vi "Z900_navX_Internal_StartLoop.vi"(8 "error in (no error)":errorcluster, 11 "navX Device":T1={"Interface"={"Protocol"=enum."SERIAL", "Update Rate (4Hz-60Hz)"=4, "navX Open TypeDef"=variant}, "Notify Packet"=refnum, "Loop VI Refnum"=refnum, "Ready to Close Occurrence Refnum"=refnum} {"Interface"."Update Rate (4Hz-60Hz)" min=4 max=60 step=1}) -> (0 "error out":errorcluster, 3 "navX Device":T1={"Interface"={"Protocol"=enum."SERIAL", "Update Rate (4Hz-60Hz)"=4, "navX Open TypeDef"=variant}, "Notify Packet"=refnum, "Loop VI Refnum"=refnum, "Ready to Close Occurrence Refnum"=refnum} {"Interface"."Update Rate (4Hz-60Hz)" min=4 max=60 step=1})   [LabVIEW 2016, in "navX Library v2.lvlib"]
doc: "This navX VI handles starting the background processing loop for the navX.\nTHIS VI SHOULD NOT BE CALLED BY THE USER!"
uses:
  navX Library v2.lvlib
  TypeDefs/Z900_navX_DeviceTypeDef.ctl
  TypeDefs/Z900_navX_ProtocolTypeDef.ctl
  TypeDefs/Z900_navX_NotifyPacketTypeDef.ctl
  TypeDefs/Z900_navX_ActionTypeDef.ctl
  Z900_navX_Internal_ProcessingLoop.vi
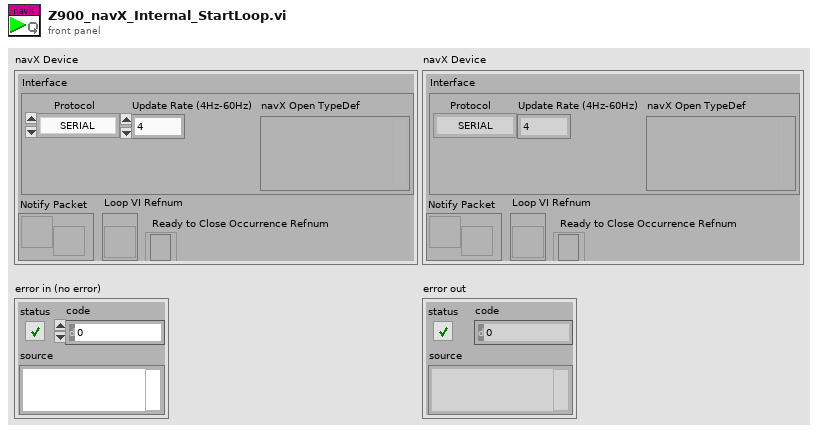
[diagram p1: front panel]
types:
  T1 = typedef "navX Library v2.lvlib/Z900_navX_DeviceTypeDef.ctl" = cluster{"Interface":cluster{"Protocol":T2, "Update Rate (4Hz-60Hz)":u8, "navX Open TypeDef":variant}, "Notify Packet":refnum<notifier>, "Loop VI Refnum":refnum<vi>, "Ready to Close Occurrence Refnum":refnum<k4>}
  T2 = typedef "navX Library v2.lvlib/Z900_navX_ProtocolTypeDef.ctl" = enum16{"SERIAL", "I2C", "SPI"}
  T3 = typedef "navX Library v2.lvlib/Z900_navX_NotifyPacketTypeDef.ctl" = cluster{"navX Action":T4, "Data":variant}
  T4 = typedef "navX Library v2.lvlib/Z900_navX_ActionTypeDef.ctl" = enum16{"None", "Halt", "Update Serial Protocol", "Zero-Yaw", "Zero-Displacement", "Zero-Velocity"}
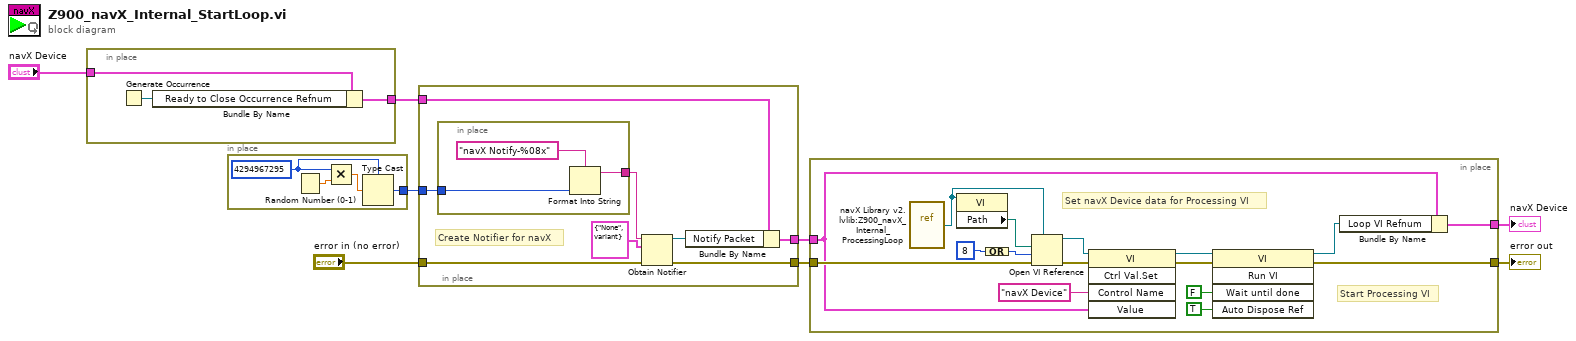
[diagram p0: block diagram]
diagram:
  n1 = in-place {
    in-place-border: "navX Device" -> [w11]
    in-place-border: [w9] -> w2
    n2 = Generate Occurrence() -> (w10:refnum<k4>)
    n3 = Bundle By Name(cluster=w11, "Ready to Close Occurrence Refnum"=w10) -> (w9:T1)
  }
  n4 = in-place {
    in-place-border: [w12] -> w8
    w14 = u32 4294967295
    n5 = Random Number (0-1)() -> (number: 0 to 1=w15:dbl)
    n6 = Multiply(x=w14, y=w15) -> (x*y=w13:dbl)
    n7 = Type Cast(type=w14, x=w13) -> (*(type *) &x=w12:u32)
  }
  n8 = in-place {
    in-place-border: w2 -> [w23]
    in-place-border: [w22] -> w5
    in-place-border: "error in (no error)" -> [w19]
    in-place-border: w8 -> [w17]
    in-place-border: [w16] -> w6
    # "Create Notifier for navX"
    n9 = in-place {
      in-place-border: [w25] -> w18
      in-place-border: w17 -> [w24]
      n10 = Format Into String(format string="navX Notify-%08x" ("name (unnamed)"), w24) -> (resulting string=w25:string)  [unwired: 2 in, 1 out]
    }
    n11 = Obtain Notifier(name (unnamed)=w18, notification data type=T3 {"navX Action"=enum."None", "Data"=variant} ("navX Notify Packet"), error in (no error)=w19) -> (notifier out=w21:refnum<notifier>, error out=w16:errorcluster)  [unwired: 1 in, 1 out]
    n12 = Bundle By Name(cluster=w23, "Notify Packet"=w21) -> (w22:T1)
  }
  n13 = in-place {
    in-place-border: w6 -> [w40]
    in-place-border: [w41] -> w4
    in-place-border: [w42] -> w3
    in-place-border: w5 -> [w39]
    # "Start Processing VI"
    # "Set navX Device data for Processing VI"
    n14 = vi-ref "navX Library v2.lvlib:Z900_navX_Internal_ProcessingLoop.vi"() -> (w28:refnum<vi>)
    n15 = property class="VI"(reference=w28) -> ("Path"=w37:path)  [unwired: 1 in, 2 out]
    n16 = Compound Arithmetic op=OR(8) -> (w38:i32)
    n17 = Open VI Reference(type specifier VI Refnum (for type only)=w28, vi path=w37, options=w38, error in (no error)=w40) -> (vi reference=w31:refnum<vi>, error out=w27:errorcluster)  [unwired: 2 in]
    n18 = invoke class="VI" method="Ctrl Val.Set"(reference=w31, error in=w27, "Control Name"="navX Device" ("format string"), "Value"=w39) -> (reference out=w33:refnum<vi>, error out=w32:errorcluster)  [unwired: 1 in, 3 out]
    n19 = invoke class="VI" method="Run VI"(reference=w33, error in=w32, "Wait until done"=FALSE ("Wait Until Done"), "Auto Dispose Ref"=TRUE ("Auto Dispose Reference")) -> (reference out=w30:refnum<vi>, error out=w42:errorcluster)  [unwired: 1 in, 3 out]
    n20 = Bundle By Name(cluster=w39, "Loop VI Refnum"=w30) -> (w41:T1)
  }
  "navX Device" <- w4
  "error out" <- w3
